vi "SR SIM921 Get Curve Header Info.vi"(4 "Error In":errorcluster, 5 "Curve #":i32, 6 "SIM Slot #":T1(radio), 7 "VISA session":refnum<visa-resource-name>) -> (0 "Error Out":errorcluster, 1 "Curve Header":T2, 3 "dup VISA session":refnum<visa-resource-name>)   [LabVIEW 2020]
doc: "This VI reads a curve header from the LakeShore Model 370 AC Resistance Bridge and returns the parsed data.\nScott Hannahs, <sth@magnet.fsu.edu> NHMFL-FSU, May 2003"
uses:
  <vilib>/regexp/Match Regular Expression.xnode
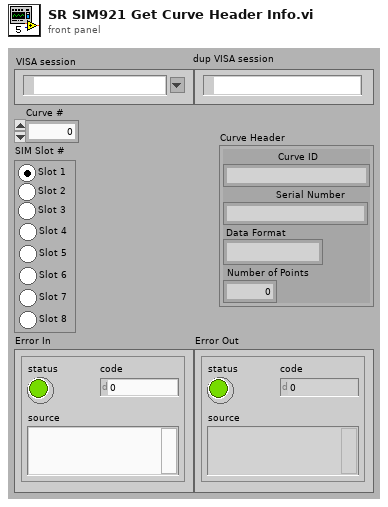
[diagram p1: front panel]
types:
  T1 = enum32{"Slot 1", "Slot 2", "Slot 3", "Slot 4", "Slot 5", "Slot 6", "Slot 7", "Slot 8"}
  T2 = cluster{"Curve ID":string, "Serial Number":string, "Data Format":string, "Number of Points":u32}
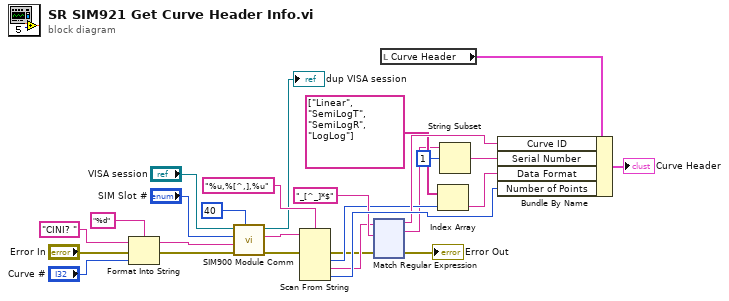
[diagram p0: block diagram]
diagram:
  n1 = Format Into String(format string="%d", initial string="CINI? " ("String to Write"), error in="Error In", "Curve #") -> (resulting string=w23:string, error out=w8:errorcluster)
  n2 = call "SIM900 Module Comm.vi"("Wait (ms)"=u32 40 ("wait (mS)"), "Error In"=w8, "Query"=w23, "Slot"="SIM Slot #", "VISA Resource Name"="VISA session") -> ("Error Out"=w7:errorcluster, "Response"=w26:string, "dup VISA Session"=→"dup VISA session":refnum<visa-resource-name>)  [unwired: 4 in]
  n3 = Scan From String(format string="%u,%[^,],%u", input string=w26, error in=w7) -> (error out=w6:errorcluster, output 1=w11:u32, output 2=w13:string, output 3=w25:u32)  [unwired: 4 in, 2 out]
  n4 = xnode "Match Regular Expression"("input string"=w13, "regular expression"="_[^_]*$", "error in"=w6) -> ("before match"=w14:string, "whole match"=w3:string, "error out"=→"Error Out":errorcluster)  [unwired: 3 in, 2 out]
  n5 = local read "Curve Header"() -> (w16:T2)
  n6 = Index Array(array=string[] ["Linear", "SemiLogT", "SemiLogR", "LogLog"], index=w11) -> (element=w10:string)
  n7 = String Subset(string=w3, offset (0)=1) -> (substring=w2:string)  [unwired: 1 in]
  n8 = Bundle By Name(cluster=w16, "Curve ID"=w14, "Serial Number"=w2, "Data Format"=w10, "Number of Points"=w25) -> (→"Curve Header":T2)
